vi "Generate RPC Messages.vi"(7 "Messages MetaData":T1[](array[typedef]), 8 "error in (no error)":errorcluster, 11 "Library":refnum<vi>) -> (0 "error out":errorcluster, 3 "Library":refnum<vi>)   [LabVIEW 2019, in "gRPC Template Creation Utility.lvlib"]
uses:
  gRPC Template Creation Utility.lvlib
  TypeDefs/Message Element Metadata (Scripting).ctl
  TypeDefs/Message Metadata (Scripting).ctl
  TypeDefs/Message Element Type.ctl
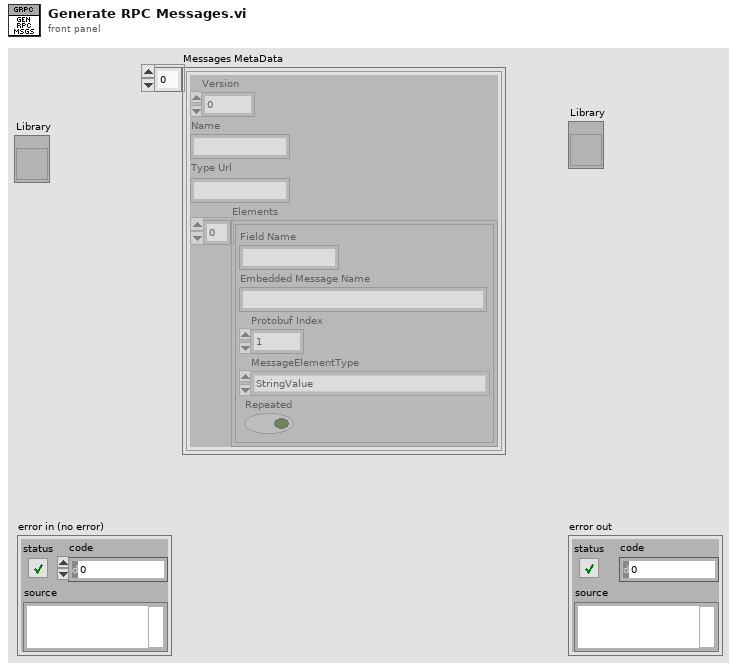
[diagram p1: front panel]
types:
  T1 = typedef "gRPC Template Creation Utility.lvlib/Message Metadata (Scripting).ctl" = cluster{"Version":i32, "Name":string, "Type Url":string, "Elements":T2[]}
  T2 = typedef "gRPC Template Creation Utility.lvlib/Message Element Metadata (Scripting).ctl" = cluster{"Field Name":string, "Embedded Message Name":string, "Protobuf Index":i32, "MessageElementType":T3, "Repeated":bool}
  T3 = typedef "gRPC Template Creation Utility.lvlib/Message Element Type.ctl" = enum32{"Int32Value", "FloatValue", "DoubleValue", "BoolValue", "StringValue", "MessageValue", "Int64Value", "UInt32Value", "UInt64Value", "EnumValue", "Bytes", "Fixed64", "Fixed32", "SFixed64", "SFixed32", "SInt64", "SInt32"}
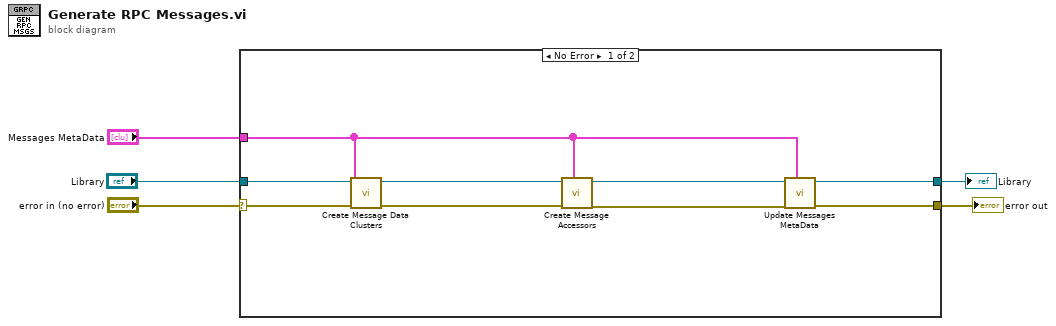
[diagram p0: block diagram]
diagram:
  n1 = case shown="No Error" "error in (no error)" {
    selector: "error in (no error)" -> [w12 w16]
    tunnel: [w11 w16] -> w5
    tunnel: [w7 w15] -> w4
    tunnel: "Messages MetaData" -> [w6 _]
    tunnel: "Library" -> [w10 w15]
    frame No Error {
      n2 = call "Create Message Data Clusters.vi"("error in (no error)"=w12, "Message parameters"=w6, "Library"=w10) -> ("error out"=w13:errorcluster, "Library"=w14:refnum<vi>)  [unwired: 7 in]
      n3 = call "Create Message Accessors.vi"("Message parameters"=w6, "error in (no error)"=w13, "Library"=w14) -> ("error out"=w9:errorcluster, "Library"=w8:refnum<vi>)  [unwired: 7 in]
      n4 = call "Update Messages MetaData.vi"("Messages MetaData"=w6, "error in (no error)"=w9, "Library"=w8) -> ("error out"=w11:errorcluster, "Library"=w7:refnum<vi>)  [unwired: 7 in]
    }
    frame Error {
    }
  }
  "error out" <- w5
  "Library" <- w4
